vi "VisBx Simulation mit Enum_PNS.vi"() -> ()   [LabVIEW 2020, in "PNS.lvlib" / "PNS Anlagenuebersicht.lvlib"]
uses:
  PNS Anlagenuebersicht.lvlib
  PNS Ventile.ctl
panel:
  out "Fehler (Ausgang)":errorcluster
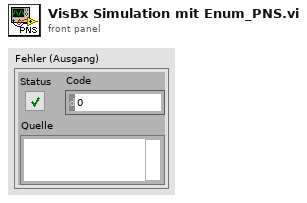
[diagram p1: front panel]
types:
  T1 = typedef "PNS.lvlib/PNS Anlagenuebersicht.lvlib/PNS Ventile.ctl" = cluster{"-Y01 Spülen ":bool, "-Y02 Lüften ":bool, "-Y03 Cal Gas":bool, "-Y04 Eingang":bool, "-Y05 Messen 01":bool, "-Y06 Messen 02":bool, "-Y07 Messen 03":bool, "-Y08 Messen 04":bool, "-Y09 Messen 05":bool, "-Y10 Messen 06":bool, "-Y11 Messen 07":bool, "-Y12 Messen 08":bool}
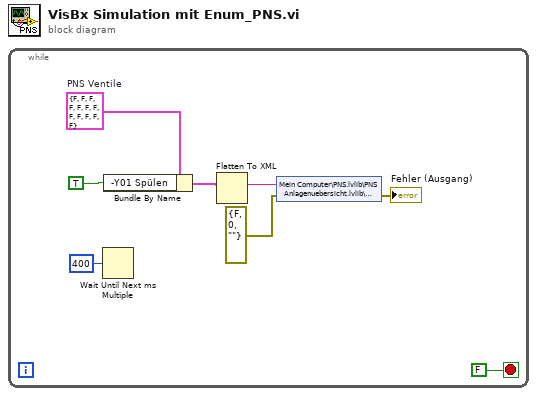
[diagram p0: block diagram]
diagram:
  n1 = while {
    stop <- FALSE stop-if-true
    w8 = T1 {"-Y01 Spülen "=FALSE, "-Y02 Lüften "=FALSE, "-Y03 Cal Gas"=FALSE, "-Y04 Eingang"=FALSE, "-Y05 Messen 01"=FALSE, "-Y06 Messen 02"=FALSE, "-Y07 Messen 03"=FALSE, "-Y08 Messen 04"=FALSE, "-Y09 Messen 05"=FALSE, "-Y10 Messen 06"=FALSE, "-Y11 Messen 07"=FALSE, "-Y12 Messen 08"=FALSE}  # PNS Ventile
    n2 = Wait Until Next ms Multiple(millisecond multiple=u32 400 ("Vielfache von ms")) -> ()  [unwired: 1 out]
    n3 = Bundle By Name(cluster=w8, "-Y01 Spülen"=TRUE) -> (w6:T1)
    n4 = Flatten To XML(6:w6) -> (2:w5:string)
    n5 = shared-variable "Mein Computer\\PNS.lvlib\\PNS Anlagenuebersicht.lvlib\\VisDat_PNS"(w5, error in=errorcluster {"status"=FALSE, "code"=0, "source"=""} ("Fehler (Eingang, kein Fehler)")) -> (error out=→"Fehler (Ausgang)":errorcluster)
  }
